vi "Concatenate all slot EEPROM arrays.vi"(8 "Error In":errorcluster, 10 "N slots occupied":i32 min=0 max=8, 11 "VISA resource name in":refnum<visa-resource-name>) -> (0 "Error out":errorcluster, 1 "ACK (all)":bool, 2 "All slot EEPROM values":T1[](array[typedef]), 3 "VISA resource name out":refnum<visa-resource-name>)   [LabVIEW 2015]
uses:
  Ctls/EEPROM page.ctl
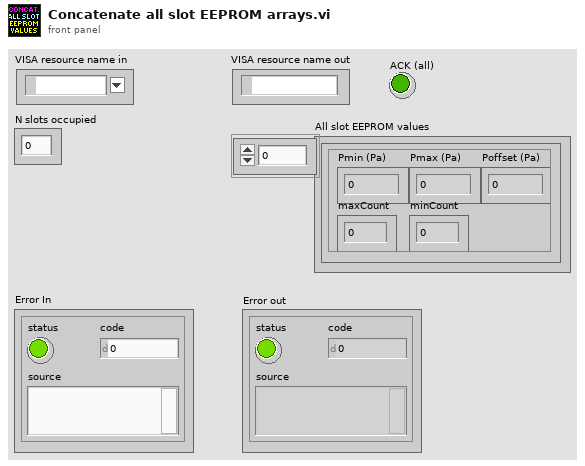
[diagram p1: front panel]
types:
  T1 = typedef "EEPROM page.ctl" = cluster{"Pmin (Pa)":sgl, "Pmax (Pa)":sgl, "maxCount":u16, "minCount":u16, "Poffset (Pa)":sgl}
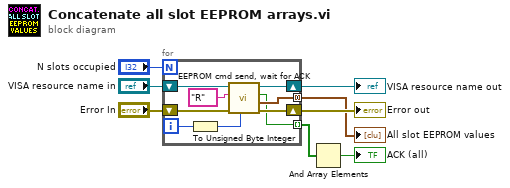
[diagram p0: block diagram]
diagram:
  n1 = for {
    N: "N slots occupied" -> [_]
    shift-right: [w16] -> w7
    shift-left: "VISA resource name in" -> [w17]
    shift-right: [w14] -> w5
    shift-left: "Error In" -> [w15]
    tunnel: [w12] -> w4 mode=concatenating
    tunnel: [w9] -> w2 mode=indexing
    i -> [w11]
    n2 = To Unsigned Byte Integer(number=w11) -> (unsigned 8bit integer=w10:u8)
    n3 = call "EEPROM cmd send, wait for ACK.vi"("Slot"=w10, "Error In"=w15, "R / W"="R", "VISA resource name in"=w17) -> ("Error out"=w14:errorcluster, "Single slot EEPROM values returned"=w12:T1[], "ACK ok"=w9:bool, "VISA resource name out"=w16:refnum<visa-resource-name>)  [unwired: 2 in]
  }
  "All slot EEPROM values" <- w4
  "VISA resource name out" <- w7
  "Error out" <- w5
  n4 = And Array Elements(Boolean array=w2) -> (logical AND=→"ACK (all)":bool)
